vi "Von Neumann Entropy.vi"(7 "QuWires Array":refnum<class "QuWire.lvclass">[](array[class])) -> (8 "Von Neumann entropy":dbl)   [LabVIEW 2020]
uses:
  QuSim/QuWire/QuWire.lvclass
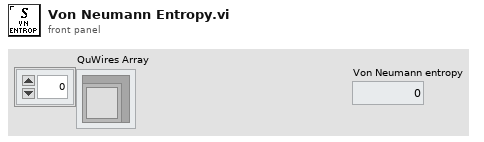
[diagram p1: front panel]
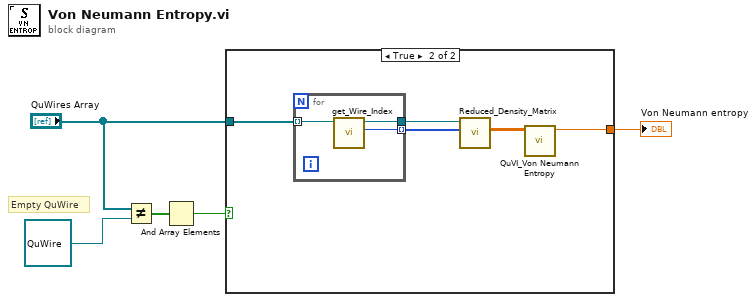
[diagram p0: block diagram]
diagram:
  # "Empty QuWire"
  n1 = Not Equal?(x="QuWires Array", y=refnum<class "QuWire.lvclass"> refnum ("QuWire in")) -> (x != y?=w4:bool[])
  n2 = And Array Elements(Boolean array=w4) -> (logical AND=w5:bool)
  n3 = case shown="True" w5 {
    tunnel: "QuWires Array" -> [_ w10]
    tunnel: [_ w6] -> w1
    frame False {
    }
    frame True {
      n4 = for {
        tunnel: w10 -> [w13] mode=indexing
        tunnel: [w12] -> w9
        tunnel: [w11] -> w8 mode=indexing
        n5 = call "get_Wire_Index.vi"("QuWire in"=w13) -> ("Wire Index"=w11:i32, "QuWire out"=w12:refnum<class "QuWire.lvclass">)  [unwired: 8 in, 1 out]
      }
      n6 = call "Reduced_Density_Matrix.vi"("Qubits to Keep"=w8, "QuWire in"=w9) -> ("Reduced Density Matrix"=w7:cdb[][])  [unwired: 6 in, 3 out]
      n7 = call "QuVI_Von Neumann Entropy.vi"("Density matrix"=w7) -> ("Von Neumann entropy"=w6:dbl)  [unwired: 10 in]
    }
  }
  "Von Neumann entropy" <- w1
